vi "readDBL.vi"(8 "error in (no error)":errorcluster, 11 "ModbusBuffer in":refnum<class "ModbusBufferBuilder.lvclass">) -> (0 "error out":errorcluster, 2 "Output":dbl, 3 "ModbusBuffer out":refnum<class "ModbusBufferBuilder.lvclass">)   [LabVIEW 2016, in "ModbusBufferBuilder.lvclass"]
uses:
  ModbusBufferBuilder.lvclass
  ModbusBufferBuilder.lvclass/ModbusBufferBuilder.ctl
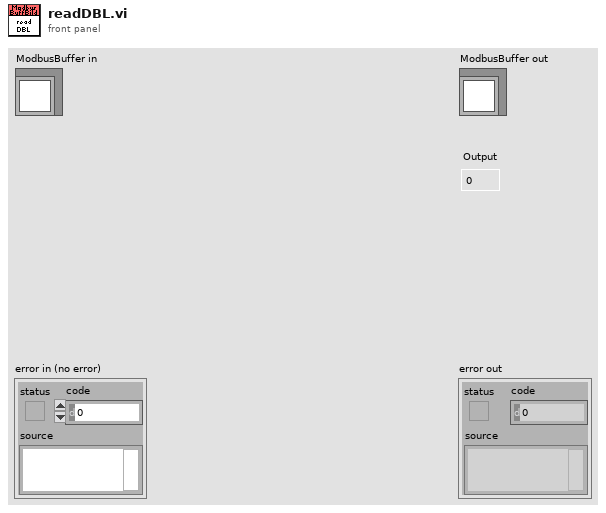
[diagram p1: front panel]
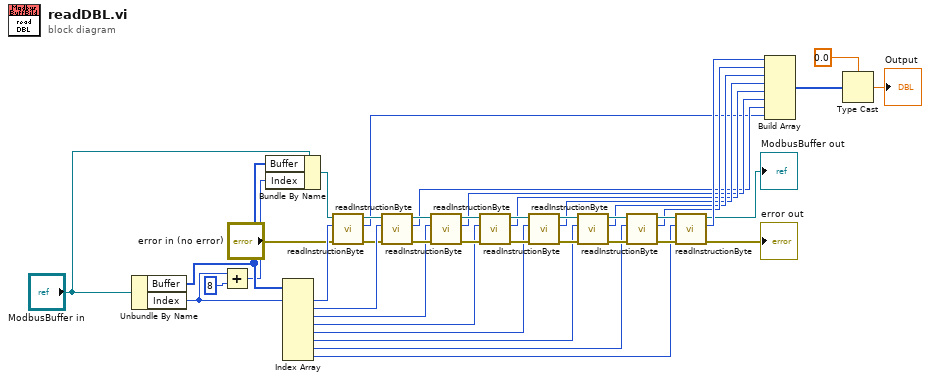
[diagram p0: block diagram]
diagram:
  n1 = Unbundle By Name("ModbusBuffer in") -> ("Buffer"=w41:u16[], "Index"=w37:i32)
  n2 = Add(x=w37, y=8) -> (x+y=w35:i32)
  n3 = Bundle By Name(cluster="ModbusBuffer in", "Buffer"=w41, "Index"=w35) -> (w39:refnum<class "ModbusBufferBuilder.lvclass">)
  n4 = Index Array(array=w41, index #1=w37) -> (element #1=w40:u16, element #2=w33:u16, element #3=w27:u16, element #4=w26:u16, element #5=w16:u16, element #6=w15:u16, element #7=w14:u16, element #8=w13:u16)  [unwired: 7 in]
  n5 = call "readInstructionByte.vi"("error in (no error)"="error in (no error)", "Instruction"=w40, "ModbusBuffer in"=w39) -> ("error out"=w32:errorcluster, "Output"=w5:u8, "ModbusBuffer out"=w34:refnum<class "ModbusBufferBuilder.lvclass">)  [unwired: 6 in]
  n6 = call "readInstructionByte.vi"("error in (no error)"=w32, "Instruction"=w33, "ModbusBuffer in"=w34) -> ("error out"=w29:errorcluster, "Output"=w6:u8, "ModbusBuffer out"=w31:refnum<class "ModbusBufferBuilder.lvclass">)  [unwired: 6 in]
  n7 = call "readInstructionByte.vi"("error in (no error)"=w29, "Instruction"=w27, "ModbusBuffer in"=w31) -> ("error out"=w28:errorcluster, "Output"=w7:u8, "ModbusBuffer out"=w30:refnum<class "ModbusBufferBuilder.lvclass">)  [unwired: 6 in]
  n8 = call "readInstructionByte.vi"("error in (no error)"=w28, "Instruction"=w26, "ModbusBuffer in"=w30) -> ("error out"=w21:errorcluster, "Output"=w8:u8, "ModbusBuffer out"=w25:refnum<class "ModbusBufferBuilder.lvclass">)  [unwired: 6 in]
  n9 = call "readInstructionByte.vi"("error in (no error)"=w21, "Instruction"=w16, "ModbusBuffer in"=w25) -> ("error out"=w20:errorcluster, "Output"=w9:u8, "ModbusBuffer out"=w24:refnum<class "ModbusBufferBuilder.lvclass">)  [unwired: 6 in]
  n10 = call "readInstructionByte.vi"("error in (no error)"=w20, "Instruction"=w15, "ModbusBuffer in"=w24) -> ("error out"=w19:errorcluster, "Output"=w10:u8, "ModbusBuffer out"=w23:refnum<class "ModbusBufferBuilder.lvclass">)  [unwired: 6 in]
  n11 = call "readInstructionByte.vi"("error in (no error)"=w19, "Instruction"=w14, "ModbusBuffer in"=w23) -> ("error out"=w18:errorcluster, "Output"=w11:u8, "ModbusBuffer out"=w22:refnum<class "ModbusBufferBuilder.lvclass">)  [unwired: 6 in]
  n12 = call "readInstructionByte.vi"("error in (no error)"=w18, "Instruction"=w13, "ModbusBuffer in"=w22) -> ("error out"=→"error out":errorcluster, "Output"=w12:u8, "ModbusBuffer out"=→"ModbusBuffer out":refnum<class "ModbusBufferBuilder.lvclass">)  [unwired: 6 in]
  n13 = Build Array(w12, w11, w10, w9, w8, w7, w6, w5) -> (w4:u8[])
  n14 = Type Cast(type=0.0, x=w4) -> (*(type *) &x=→"Output":dbl)
